vi "Set Tasks.vi"(8 "error in (no error)":errorcluster, 10 "Tasks":map{string, refnum<class "Task Base.lvclass">}(c390), 11 "Study Base in":refnum<class "Study Base.lvclass">) -> (0 "error out":errorcluster, 3 "Study Base out":refnum<class "Study Base.lvclass">)   [LabVIEW 2023, in "HAL GOOP4.lvlib" / "Study Base.lvclass"]
uses:
  Study Base.lvclass
  Task Base/Task Base.lvclass
  Study Base.lvclass/Study Base.ctl
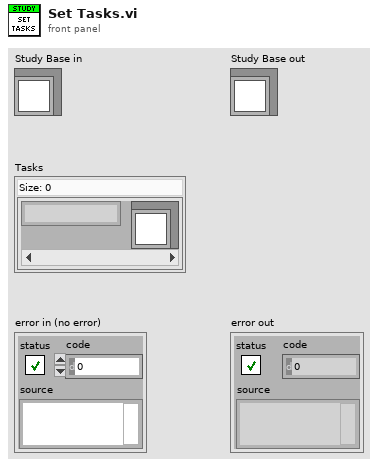
[diagram p1: front panel]
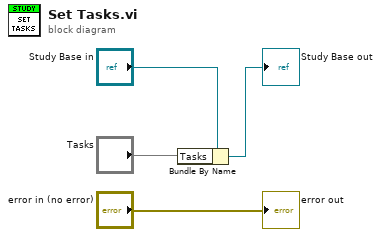
[diagram p0: block diagram]
diagram:
  n1 = Bundle By Name(cluster="Study Base in", "Tasks"="Tasks") -> (→"Study Base out":refnum<class "Study Base.lvclass">)
  "error out" <- "error in (no error)"
